vi "Odometry.vi"(1 "error in":errorcluster, 3 "node":string) -> (0 "error out":errorcluster, 4 "Odometry":T1)   [LabVIEW 2012]
doc: "Reads in the odometry from the Turtlebot"
uses:
  ROS/Code/SubVIs/_ROSDirection.ctl
  ROS/Code/Console/Servers/ServerSubs/TopicDef.ctl
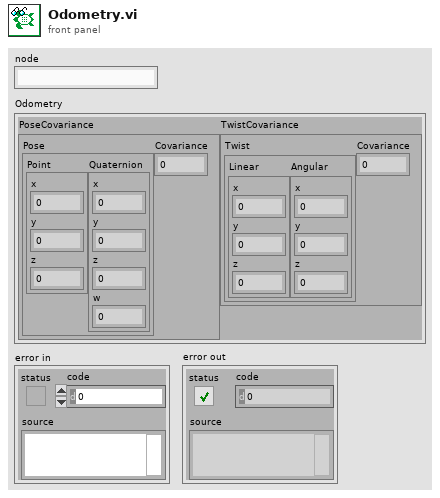
[diagram p1: front panel]
types:
  T1 = cluster{"PoseCovariance":cluster{"Pose":cluster{"Point":cluster{"x":dbl, "y":dbl, "z":dbl}, "Quaternion":cluster{"x":dbl, "y":dbl, "z":dbl, "w":dbl}}, "Covariance":dbl}, "TwistCovariance":cluster{"Twist":cluster{"Linear":cluster{"x":dbl, "y":dbl, "z":dbl}, "Angular":cluster{"x":dbl, "y":dbl, "z":dbl}}, "Covariance":dbl}}
  T2 = typedef "TopicDef.ctl" = cluster{"Topic":string, "Type":string, "Action":T3, "Update (ms)":u16, "queue size":u16}
  T3 = typedef "_ROSDirection.ctl" = enum16{"Node", "Publisher", "Subscriber", "ServiceClient", "ServiceProvider"}
  T4 = typedef "_ROSControl.ctl" = cluster{"topic port":u16, "Node":string, "topic":string, "type":string, "node port":u16, "error ":errorcluster, "Direction":T3, "Update (ms)":u16, "FIFO size":u16}
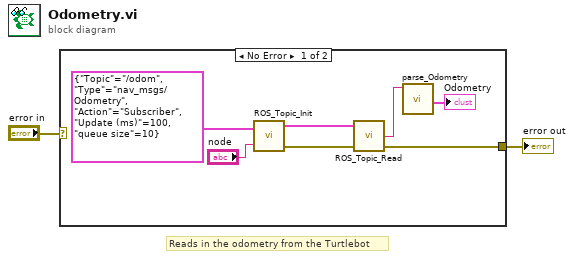
[diagram p0: block diagram]
diagram:
  # "Reads in the odometry from the Turtlebot"
  n1 = case shown="No Error" "error in" {
    selector: "error in" -> [_ w10]
    tunnel: [w6 w10] -> w1
    frame No Error {
      n2 = call "ROS_Topic_Init.vi"("Definitions"=T2 {"Topic"="/odom", "Type"="nav_msgs/Odometry", "Action"=enum."Subscriber", "Update (ms)"=100, "queue size"=10}, "node"="node") -> ("ROS out"=w8:T4, "error out"=w7:errorcluster)  [unwired: 1 in]
      n3 = call "ROS_Topic_Read.vi"("error in (no error)"=w7, "ROS in"=w8) -> ("error out"=w6:errorcluster, "Reply"=w5:string)  [unwired: 1 in, 1 out]
      n4 = call "parse_Odometry.vi"("msg in"=w5) -> ("Odometry"=→"Odometry":T1)  [unwired: 4 in, 4 out]
    }
    frame Error {
    }
  }
  "error out" <- w1
